vi "mod_align TX and RX bit sequence.vi"(0 "TX Bit Sequence":i8[](array[numeric]), 5 "RX Bit Sequence":i8[](array[numeric]), 7 "# Bits removed":i32, 11 "Reset":bool) -> (4 "Aligned array":i8[](array[numeric]))   [LabVIEW 2020, in "niDMT.lvlib"]
uses:
  <vilib>/addons/Modulation/niDMT.lvlib
panel:
  # "This VI removes a user specified number\nof bits from the TX Bit Sequence and returns\na sequence that is aligned with the RX Bit\nSequence."
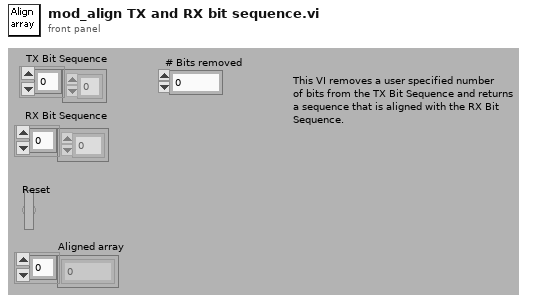
[diagram p1: front panel]
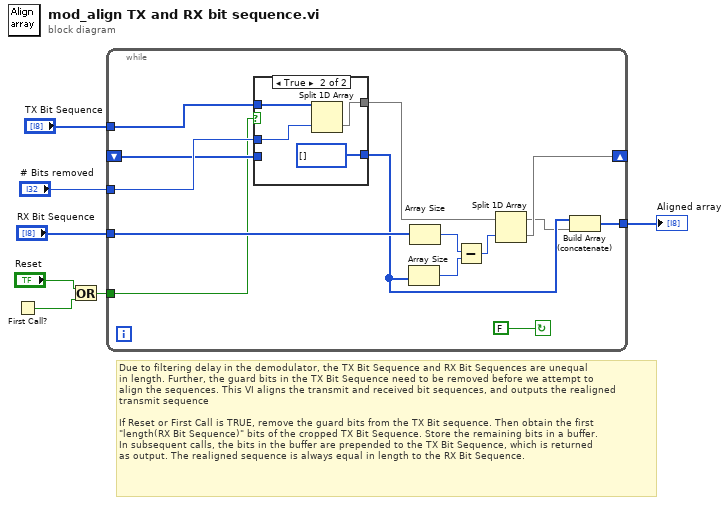
[diagram p0: block diagram]
diagram:
  # "Due to filtering delay in the demodulator, the TX Bit Sequence and RX Bit Sequences are unequal \nin length. Further, the guard bits in the TX Bit Sequence need to be removed before we attempt to \nalign the sequences. This VI aligns the transmit and received bit sequences, and outputs the realigned \ntransmit sequence\n\nIf Reset or First Call is TRUE, remove the guard bits from the TX Bit sequence. Then obtain the first\n\"length(RX Bit Sequence)\" bits of the cropped TX Bit Sequence. Store the remaining bits in a buffer.\nIn subsequent calls, the bits in the buffer are prepended to the TX Bit Sequence, which is returned\nas output. The realigned sequence is always equal in length to the RX Bit Sequence."
  n1 = First Call?() -> (First Call?: T/F=w6:bool)
  n2 = Or(x="Reset", y=w6) -> (x .or. y?=w2:bool)
  n3 = while {
    tunnel: "TX Bit Sequence" -> [w21]
    tunnel: "# Bits removed" -> [w20]
    tunnel: "RX Bit Sequence" -> [w18]
    shift-right: [w11] -> _
    shift-left: _ -> [w13]
    tunnel: w2 -> [w12]
    tunnel: [w8] -> w1
    stop <- FALSE continue-if-true
    n4 = case shown="True" w12 {
      tunnel: w21 -> [w23 w27]
      tunnel: w20 -> [_ w26]
      tunnel: [w23 w25] -> w19
      tunnel: w13 -> [w22 _]
      tunnel: [w22 i8[] [] ("t")] -> w10
      frame False {
      }
      frame True {
        n5 = Split 1D Array(array=w27, index=w26) -> (second subarray=w25:i8[])  [unwired: 1 out]
      }
    }
    n6 = Array Size(array=w10) -> (size(s)=w16:i32)
    n7 = Array Size(array=w18) -> (size(s)=w17:i32)
    n8 = Subtract(x=w17, y=w16) -> (x-y=w15:i32)
    n9 = Split 1D Array(array=w19, index=w15) -> (first subarray=w9:i8[], second subarray=w11:i8[])
    n10 = Build Array (concatenate)(w10, w9) -> (w8:i8[])
  }
  "Aligned array" <- w1
